vi "Post Process Count Convert.vi"(0 "pInputImage":i32, 1 "iBaseline":i32, 2 "iEmGain":i32, 3 "fSensitivity":sgl, 5 "pOutputImage":i32, 7 "iOutputBufferSize":i32, 9 "iNumImages":i32, 10 "iWidth":i32, 12 "iMode":i32, 13 "fQE":sgl, 14 "iHeight":i32) -> (4 "pInputImage out":i32, 6 "pOutputImage out":i32, 8 "function return":u32)   [LabVIEW 2018, in "AndorSDK.lvlib"]
doc: "EXPNETTYPE unsigned int WINAPI PostProcessCountConvert(at_32 * pInputImage, at_32 * pOutputImage, int iOutputBufferSize, int iNumImages, int iBaseline, int iMode, int iEmGain, float fQE, float fSensitivity, int iHeight, int iWidth);"
uses:
  AndorSDK.lvlib
  ATMCD32D.dll
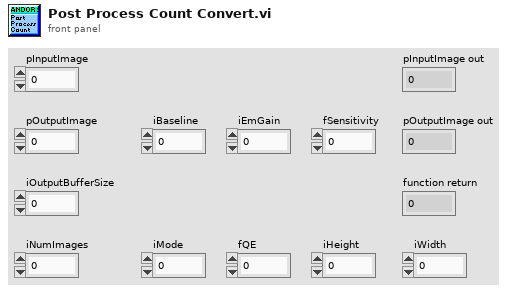
[diagram p1: front panel]
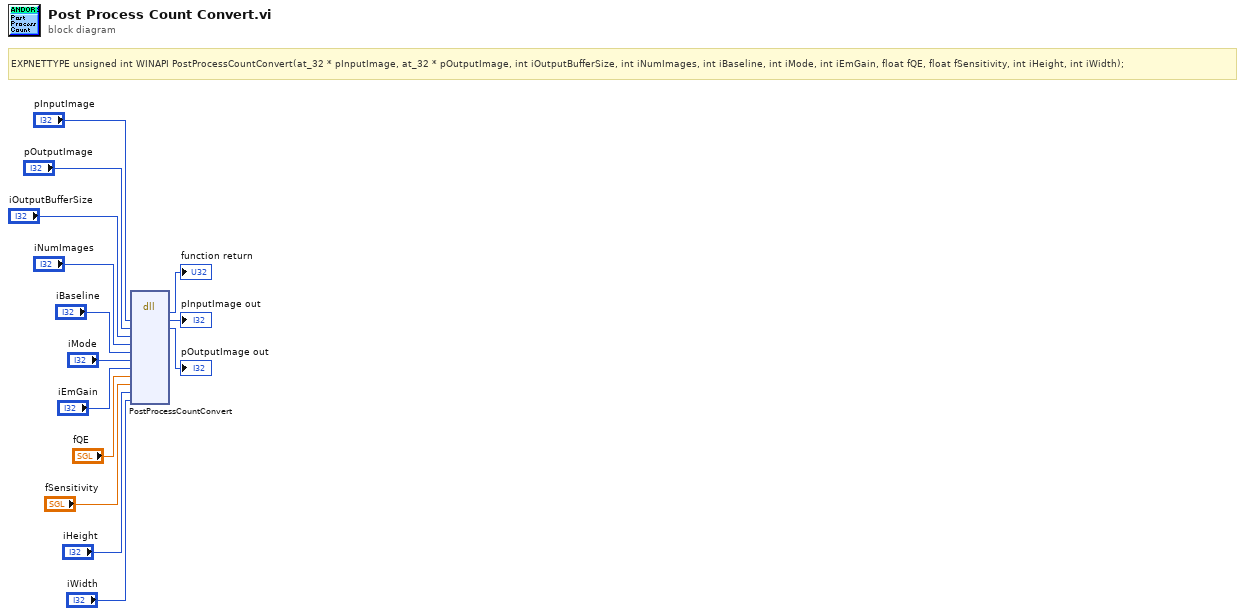
[diagram p0: block diagram]
diagram:
  # "EXPNETTYPE unsigned int WINAPI PostProcessCountConvert(at_32 * pInputImage, at_32 * pOutputImage, int iOutputBufferSize, int iNumImages, int iBaseline, int iMode, int iEmGain, float fQE, float fSensitivity, int iHeight, int iWidth);"
  n1 = dll-call lib="PTH2babs E\nPersönliches02 - Arbeit03-HiwijobsLabviewCodelibANDOR\tAndor SDK\nATMCD32D.*" fn="PostProcessCountConvert"("pInputImage"="pInputImage", "pOutputImage"="pOutputImage", "iOutputBufferSize"="iOutputBufferSize", "iNumImages"="iNumImages", "iBaseline"="iBaseline", "iMode"="iMode", "iEmGain"="iEmGain", "fQE"="fQE", "fSensitivity"="fSensitivity", "iHeight"="iHeight", "iWidth"="iWidth") -> (→"function return":u32, "pInputImage"=→"pInputImage out":i32, "pOutputImage"=→"pOutputImage out":i32)  [unwired: 12 in, 2 out]
